vi "Update Configuration Command.vi"(8 "error in":errorcluster, 10 "Config JSON":string, 11 "CoreOOB_Rx in":refnum<class "CIFCoreOOB_Rx.lvclass">) -> (0 "error out":errorcluster, 3 "CoreOOB_Rx out":refnum<class "CIFCoreOOB_Rx.lvclass">)   [LabVIEW 2021, in "CIFCoreOOB_Rx.lvclass"]
uses:
  CIFCoreOOB_Rx.lvclass
  D:/dev/CIF-LVCore/src/CIFUtilities/CIFOutOfBand/CIFOutOfBand.lvclass
  CIFUtilities/CIFOutOfBand/CIFOutOfBand.lvclass/CIFOutOfBand.ctl
  Typedef/OOB Core Commands.ctl
  Typedef/Template Payload.ctl
  Typedef/Channel Connection Data.ctl
  Typedef/Channel Fault Data.ctl
  CIFCoreOOB_Rx.lvclass/CIFCoreOOB_Rx.ctl
  CIFUtilities/CIFOutOfBand/CIFOutOfBand.lvclass
  <vilib>/addons/_JKI.lib/Serialization/JSON/JKI JSON Serialization.lvlib
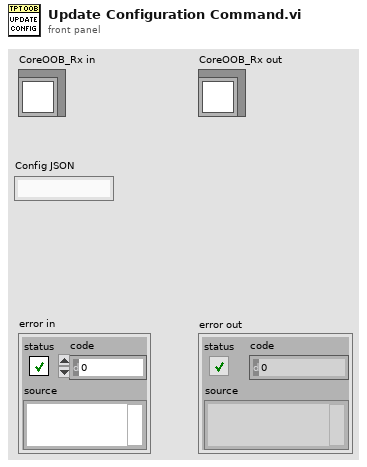
[diagram p1: front panel]
types:
  T1 = typedef "CIFCoreOOB_Rx.lvclass/OOB Core Commands.ctl" = enum8{"Start", "Pause", "Stop", "RefreshStats", "UpdateConfig", "Connect Channel", "Force Channel"}
  T2 = typedef "CIFCoreOOB_Rx.lvclass/Template Payload.ctl" = cluster{"Config Data":variant, "Connections":T3[], "Forces":T4[]}
  T3 = typedef "CIFCoreOOB_Rx.lvclass/Channel Connection Data.ctl" = cluster{"Publisher Name":string, "Subscriber Name":string, "Connection Data":u8[]}
  T4 = typedef "CIFCoreOOB_Rx.lvclass/Channel Fault Data.ctl" = cluster{"Channel Name":string, "Force Data":u8[], "Force Active":bool}
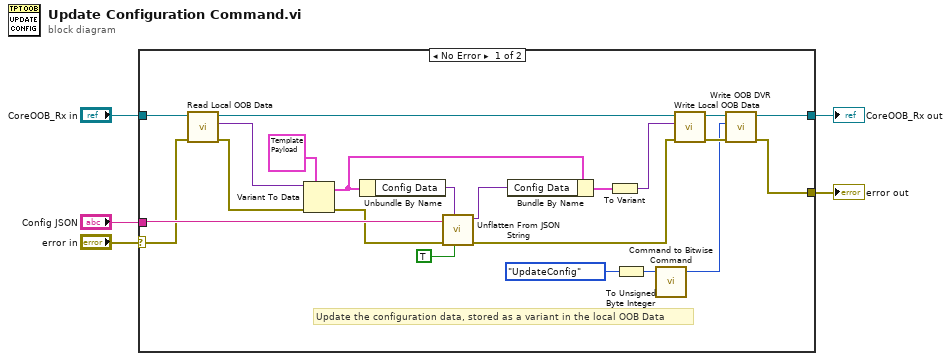
[diagram p0: block diagram]
diagram:
  n1 = case shown="No Error" "error in" {
    selector: "error in" -> [w19 w29]
    tunnel: [w26 w29] -> w4
    tunnel: "CoreOOB_Rx in" -> [w21 w28]
    tunnel: [w27 w28] -> w2
    tunnel: "Config JSON" -> [w25 _]
    frame No Error {
      # "Update the configuration data, stored as a variant in the local OOB Data"
      n2 = call "Read Local OOB Data.vi"("error in"=w19, "OOB in"=w21) -> ("error out"=w14:errorcluster, "Local OOB Data"=w18:variant, "OOB out"=w20:refnum<class "CIFCoreOOB_Rx.lvclass">)  [unwired: 7 in]
      n3 = Variant To Data(error in=w14, type=T2 {"Config Data"=variant, "Connections"=[], "Forces"=[]} ("Template Payload"), Variant=w18) -> (data=w15:T2, error out=w13:errorcluster)
      n4 = Unbundle By Name(w15) -> ("Config Data"=w16:variant)
      n5 = call <vilib>:"Unflatten From JSON String.vi"("Nulls as Defaults (F)"=TRUE, "Type and Defaults"=w16, "error in (no error)"=w13, "JSON String"=w25) -> ("error out"=w24:errorcluster, "Variant"=w23:variant)  [unwired: 6 in]
      n6 = Bundle By Name(cluster=w15, "Config Data"=w23) -> (w8:T2)
      n7 = To Variant(anything=w8) -> (Variant=w7:variant)
      n8 = To Unsigned Byte Integer(number=OOB_Core_Commands."UpdateConfig" ("OOB Main Commands")) -> (unsigned 8bit integer=w10:u8)
      n9 = call "Command to Bitwise Command.vi"("OOB Command"=w10) -> ("bit command"=w6:u64)  [unwired: 3 in]
      n10 = call "Write Local OOB Data.vi"("error in"=w24, "Local OOB Data"=w7, "OOB in"=w20) -> ("error out"=w12:errorcluster, "OOB out"=w11:refnum<class "CIFCoreOOB_Rx.lvclass">)  [unwired: 7 in]
      n11 = call "Write OOB DVR.vi"("error in"=w12, "Commands (bitwise)"=w6, "OOB in"=w11) -> ("error out"=w26:errorcluster, "OOB out"=w27:refnum<class "CIFCoreOOB_Rx.lvclass">)  [unwired: 7 in]
    }
    frame Error {
    }
  }
  "error out" <- w4
  "CoreOOB_Rx out" <- w2
